vi "Script Loaded.vi"(8 "error in (no error)":errorcluster, 11 "gScript Interpreter in":refnum<class "gScript Interpreter.lvclass">) -> (0 "error out":errorcluster, 2 "Script Loaded?":bool, 3 "gScript Interpreter out":refnum<class "gScript Interpreter.lvclass">)   [LabVIEW 2017, in "gScript Interpreter.lvclass"]
uses:
  gScript Interpreter.lvclass
  gScript Interpreter.lvclass/gScript Interpreter.ctl
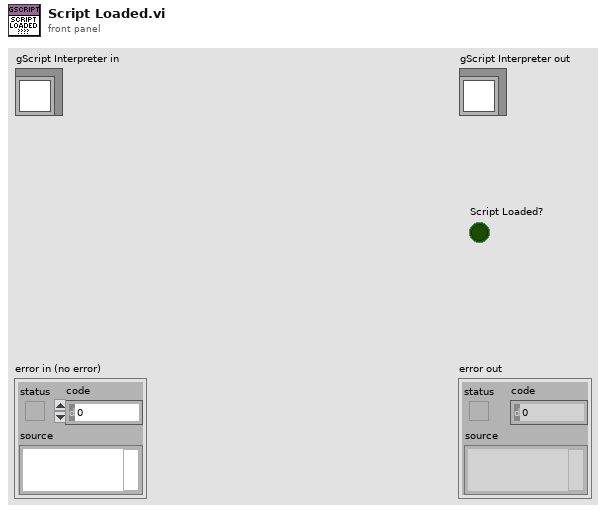
[diagram p1: front panel]
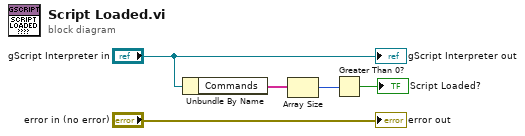
[diagram p0: block diagram]
diagram:
  n1 = Unbundle By Name("gScript Interpreter in") -> ("Commands"=w2:string[])
  n2 = Array Size(array=w2) -> (size(s)=w1:i32)
  n3 = Greater Than 0?(x=w1) -> (x > 0?=→"Script Loaded?":bool)
  "error out" <- "error in (no error)"
  "gScript Interpreter out" <- "gScript Interpreter in"
